vi "Memory.Pointer.Bounds Check.Subset.vi"(8 "error in (no error)":errorcluster, 9 "length":i64 format="%d bytes", 10 "offset":i64 format="%d bytes", 11 "Pointer in":refnum<class "Memory.Pointer.lvclass">) -> (0 "error out":errorcluster, 1 "length out":i64 format="%d bytes", 2 "offset out":i64 format="%d bytes", 3 "Pointer out":refnum<class "Memory.Pointer.lvclass">, 5 "subset valid":bool)   [LabVIEW 2016, in "LabVIEW Memory Manager.lvlib" / "Memory.Pointer.lvclass"]
uses:
  Memory.Pointer.lvclass
  Memory.Pointer.lvclass/Memory.Pointer.ctl
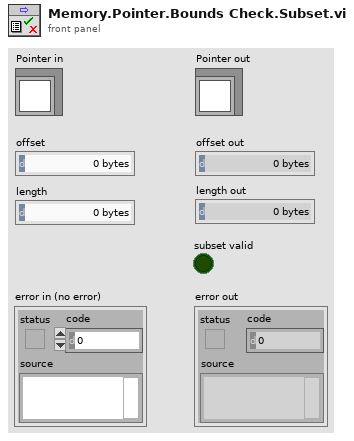
[diagram p1: front panel]
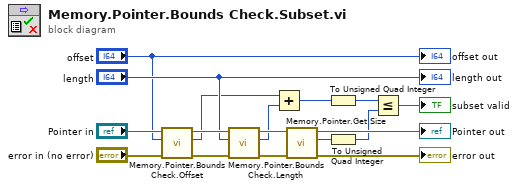
[diagram p0: block diagram]
diagram:
  n1 = call "Memory.Pointer.Bounds Check.Offset.vi"("error in (no error)"="error in (no error)", "offset"="offset", "Pointer in"="Pointer in") -> ("error out"=w4:errorcluster, "offset out"=w2:i64, "Pointer out"=w5:refnum<class "Memory.Pointer.lvclass">)  [unwired: 5 in, 1 out]
  n2 = call "Memory.Pointer.Bounds Check.Length.vi"("error in (no error)"=w4, "length"="length", "Pointer in"=w5) -> ("error out"=w10:errorcluster, "length out"=w9:i64, "Pointer out"=w11:refnum<class "Memory.Pointer.lvclass">)  [unwired: 5 in, 1 out]
  n3 = Add(x=w2, y=w9) -> (x+y=w15:i64)
  n4 = call "Memory.Pointer.Get Size.vi"("error in (no error)"=w10, "Pointer in"=w11) -> ("error out"=→"error out":errorcluster, "size"=w16:i64, "Pointer out"=→"Pointer out":refnum<class "Memory.Pointer.lvclass">)  [unwired: 7 in]
  n5 = To Unsigned Quad Integer(1:w15) -> (0:w8:u64)
  n6 = To Unsigned Quad Integer(1:w16) -> (0:w13:u64)
  n7 = Less Or Equal?(x=w8, y=w13) -> (x <= y?=→"subset valid":bool)
  "length out" <- "length"
  "offset out" <- "offset"
